vi "write TBM configuration.vi"(8 "error in":errorcluster, 10 "configuration":refnum<class "TBM configuration.lvclass">, 11 "Logic Sequencer editor node in":refnum<class "Logic Sequencer editor node.lvclass">) -> (0 "error out":errorcluster, 3 "Logic Sequencer editor node out":refnum<class "Logic Sequencer editor node.lvclass">)   [LabVIEW 2013, in "Logic Sequencer editor node.lvclass"]
uses:
  Logic Sequencer editor node.lvclass
  <vilib>/NI/Tag Bus Module Framework/root configuration/TBM configuration.lvclass
  module/configuration/Logic Sequencer configuration.lvclass
  Logic Sequencer editor node.lvclass/Logic Sequencer editor node.ctl
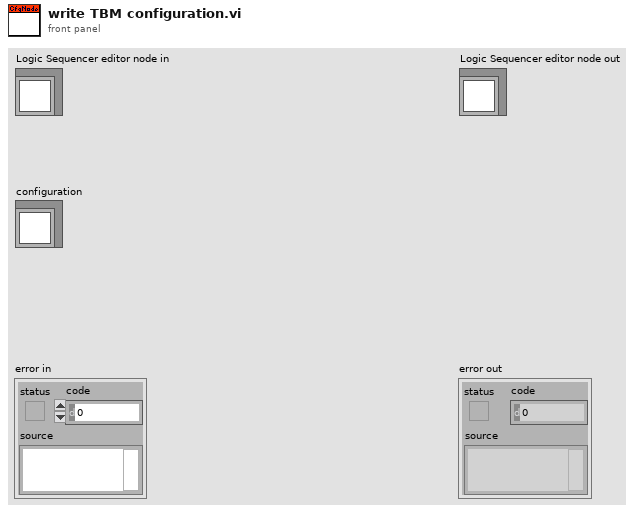
[diagram p1: front panel]
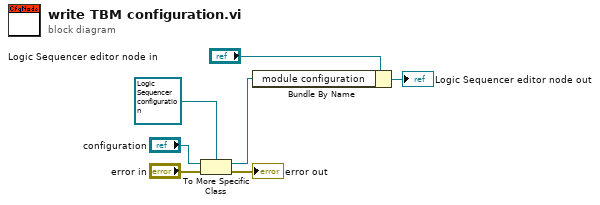
[diagram p0: block diagram]
diagram:
  n1 = To More Specific Class(target class=refnum<class "Logic Sequencer configuration.lvclass"> refnum ("module configuration"), reference="configuration", error in="error in") -> (specific class reference=w3:refnum<class "Logic Sequencer configuration.lvclass">, error out=→"error out":errorcluster)
  n2 = Bundle By Name(cluster="Logic Sequencer editor node in", "module configuration"=w3) -> (→"Logic Sequencer editor node out":refnum<class "Logic Sequencer editor node.lvclass">)
